vi "Get ProgReturn Info.vi"(11 "String":string="$AGENT.81,C8.C8,S*03") -> (1 "Chk OK or Fail":bool, 2 "Format Status":string, 3 "´¹¤ùID":string)   [LabVIEW 2019]
panel:
  in  "ToolString Input":string="$AGENT,53,VS-62U009+VS-69W014*71"
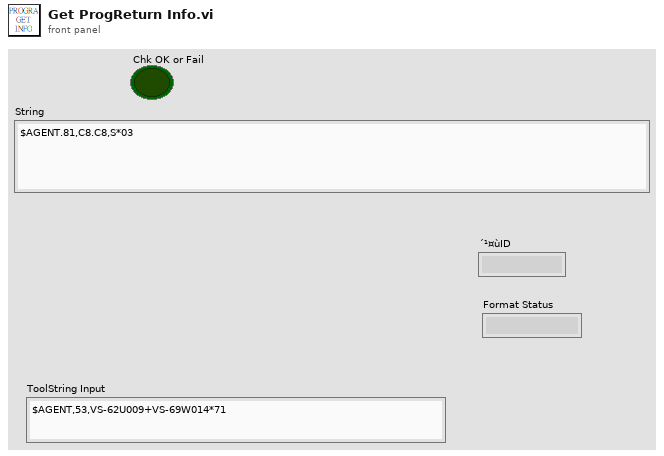
[diagram p1: front panel]
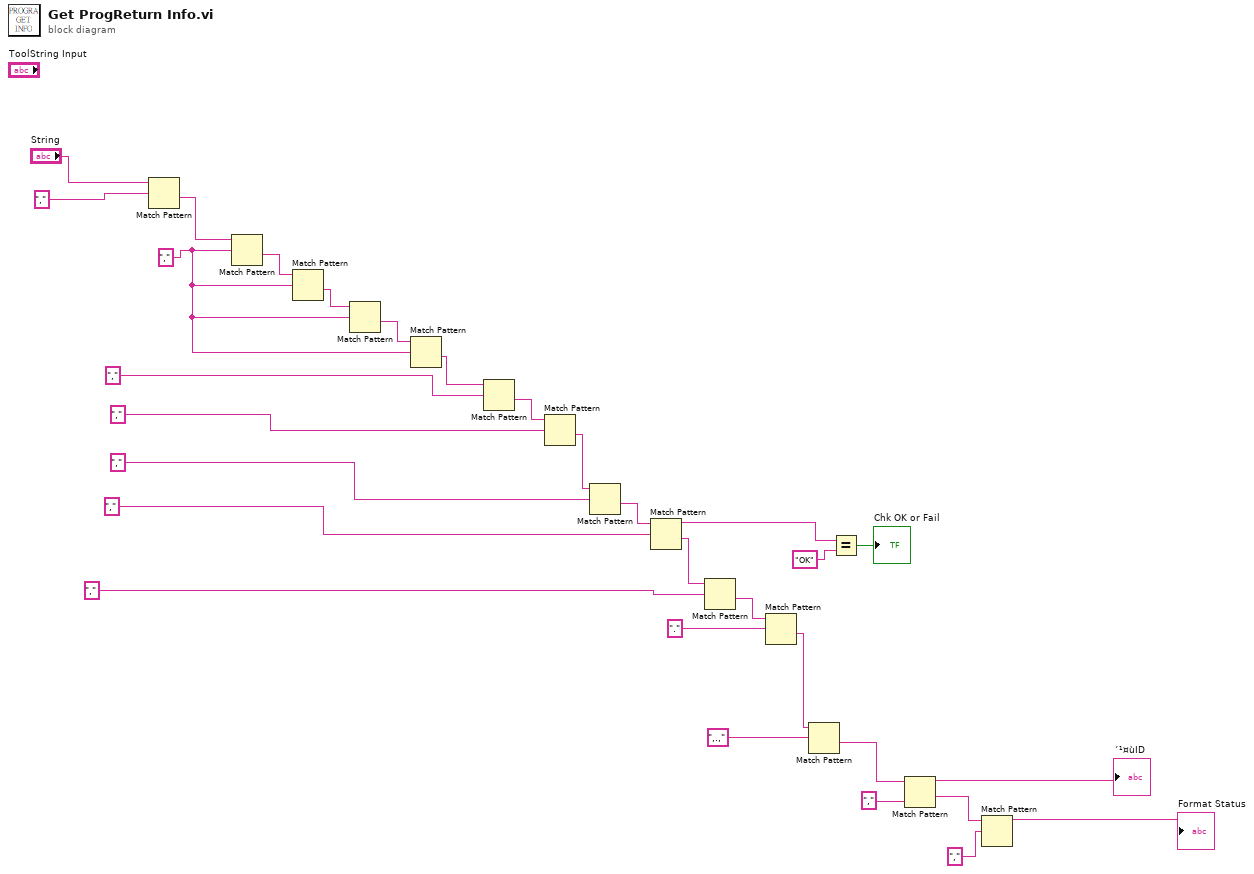
[diagram p0: block diagram]
diagram:
  w5 = ","
  n1 = Match Pattern(string="String", regular expression=",") -> (after substring=w29:string)  [unwired: 1 in, 3 out]
  n2 = Match Pattern(string=w29, regular expression=w5) -> (after substring=w28:string)  [unwired: 1 in, 3 out]
  n3 = Match Pattern(string=w28, regular expression=w5) -> (after substring=w12:string)  [unwired: 1 in, 3 out]
  n4 = Match Pattern(string=w12, regular expression=w5) -> (after substring=w26:string)  [unwired: 1 in, 3 out]
  n5 = Match Pattern(string=w26, regular expression=w5) -> (after substring=w16:string)  [unwired: 1 in, 3 out]
  n6 = Match Pattern(string=w16, regular expression=",") -> (after substring=w24:string)  [unwired: 1 in, 3 out]
  n7 = Match Pattern(string=w24, regular expression=",") -> (after substring=w15:string)  [unwired: 1 in, 3 out]
  n8 = Match Pattern(string=w15, regular expression=",") -> (after substring=w4:string)  [unwired: 1 in, 3 out]
  n9 = Match Pattern(string=w4, regular expression=",") -> (before substring=w3:string, after substring=w14:string)  [unwired: 1 in, 2 out]
  n10 = Match Pattern(string=w14, regular expression=",") -> (after substring=w19:string)  [unwired: 1 in, 3 out]
  n11 = Match Pattern(string=w19, regular expression=".") -> (after substring=w13:string)  [unwired: 1 in, 3 out]
  n12 = Match Pattern(string=w13, regular expression=",.,") -> (after substring=w10:string)  [unwired: 1 in, 3 out]
  n13 = Equal?(x=w3, y="OK") -> (x = y?=→"Chk OK or Fail":bool)
  n14 = Match Pattern(string=w10, regular expression=",") -> (before substring=→"´¹¤ùID":string, after substring=w9:string)  [unwired: 1 in, 2 out]
  n15 = Match Pattern(string=w9, regular expression=",") -> (before substring=→"Format Status":string)  [unwired: 1 in, 3 out]
